vi "NXT-Cam-Direct.vi"() -> ()   [LabVIEW 2009]
uses:
  <vilib>/NXT/Block Support/NXT_InputPort.ctl
  <vilib>/NXT/Subs/LVHSConnector.ctl
panel:
  out "Status (boolean)":bool
  out "Y Lower Right":u8
  out "X Lower Right":u8
  out "Y Upper Left":u8
  out "X Upper Left":u8
  out "Color":u8
  out "Total Tracked Objects":u8
  in  "Object Number to Track":u8 format="%x"
  in  "Tracking Mode":u8(ring)=1 items=["Disable Tracking", "Get First Object", "Get n th Object", "Enable Tracking", "Sort Objects  by size", "Sort Objects  by Colors", "Illumination on ", "Illumination Off", "Write Colormap", "Read Colormap", "Line tracking mode", "Object Tracking mode"]
  out "NXT dup":T1={"error"={"status"=FALSE, "code"=0, "source"=""}, "address"="USB0::0x0694::0x0002::001653FF017B::RAW", "NXT #"=0, "Show Error"=TRUE}
  in  "NXT":T1={"error"={"status"=FALSE, "code"=0, "source"=""}, "address"="", "NXT #"=-1, "Show Error"=TRUE}
  in  "Input Port":T2 items=["Port 1", "Port 2", "Port 3", "Port 4"]
  in  "stop Tracking":bool=TRUE
  # "mindsensors.com\nCopyright (c) 2009 by mindsensors.com\nEmail: info (<at>) mindsensors (<dot>) com\n\nThis program is free software. You can redistribute it and/or modify\nit under the terms of the GNU General Public License as published by\nthe Free Software Foundation; version 3 of the License.\nRead the license at: http://www.gnu.org/licenses/gpl.txt"
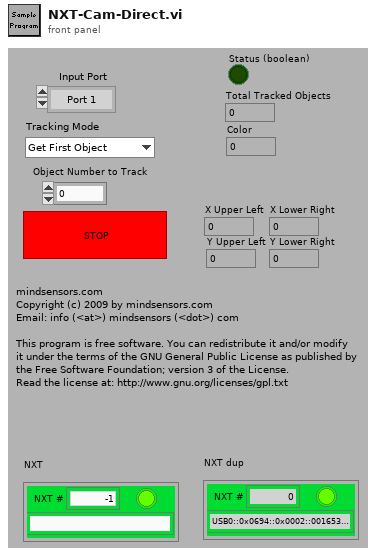
[diagram p1: front panel]
types:
  T1 = typedef "LVHSConnector.ctl" = cluster{"error":errorcluster, "address":string, "NXT #":i32, "Show Error":bool}
  T2 = typedef "NXT_InputPort.ctl" = u8
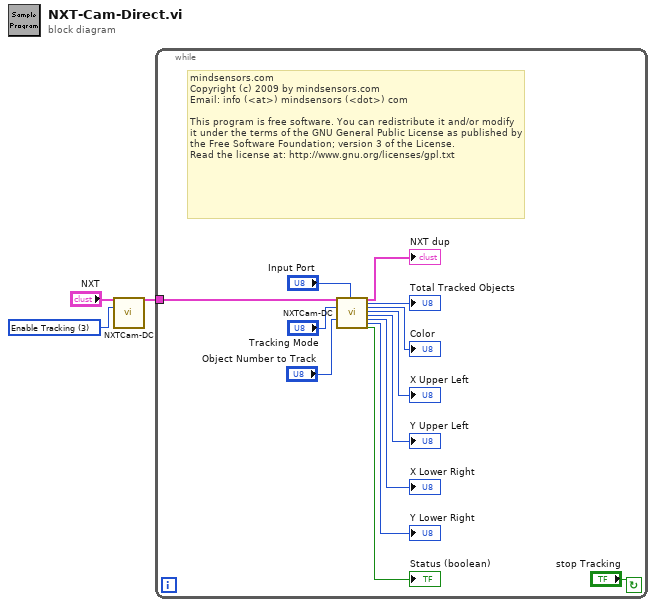
[diagram p0: block diagram]
diagram:
  w3 = u8 3 items=["Disable Tracking", "Get First Object", "Get n th Object", "Enable Tracking", "Sort Objects  by size", "Sort Objects  by Colors", "Illumination on ", "Illumination Off", "Write Colormap", "Read Colormap", "Line tracking mode", "Object Tracking mode"] ("Tracking Mode")
  n1 = call "NXTCam-DC.vi"("NXT"="NXT", "Tracking Mode"=w3) -> ("NXT dup"=w1:T1)  [unwired: 18 in, 7 out]
  n2 = while {
    tunnel: w1 -> [w14]
    stop <- "stop Tracking" continue-if-true
    # "mindsensors.com\nCopyright (c) 2009 by mindsensors.com\nEmail: info (<at>) mindsensors (<dot>) com\n\nThis program is free software. You can redistribute it and/or modify\nit under the terms of the GNU General Public License as published by\nthe Free Software Foundation; version 3 of the License.\nRead the license at: http://www.gnu.org/licenses/gpl.txt"
    n3 = call "NXTCam-DC.vi"("NXT"=w14, "Tracking Mode"="Tracking Mode", "Object Number to Track"="Object Number to Track", "Input Port"="Input Port") -> ("NXT dup"=→"NXT dup":T1, "Total Tracked Objects"=→"Total Tracked Objects":u8, "Color"=→"Color":u8, "X Upper Left"=→"X Upper Left":u8, "Y Upper Left"=→"Y Upper Left":u8, "X Lower Right"=→"X Lower Right":u8, "Y Lower Right"=→"Y Lower Right":u8, "Status (boolean)"=→"Status (boolean)":bool)  [unwired: 16 in]
  }
